vi "Read Global Header.vi"(8 "error in (no error)":errorcluster, 11 "pcap Parse and Build in":refnum<class "pcap Parse and Build.lvclass">) -> (0 "error out":errorcluster, 2 "Global Header":T1={"magic number"=2712812621, "Major Version"=2, "Minor Version"=4, "This Zone"=0, "Accuracy"=0, "Max Length"=65535, "Data Link"=1} {"magic number" format="%.0x"}, 3 "pcap Parse and Build out":refnum<class "pcap Parse and Build.lvclass">)   [LabVIEW 2021, in "pcap Parse and Build.lvclass"]
uses:
  pcap Parse and Build.lvclass
  Typedef/Global Header.ctl
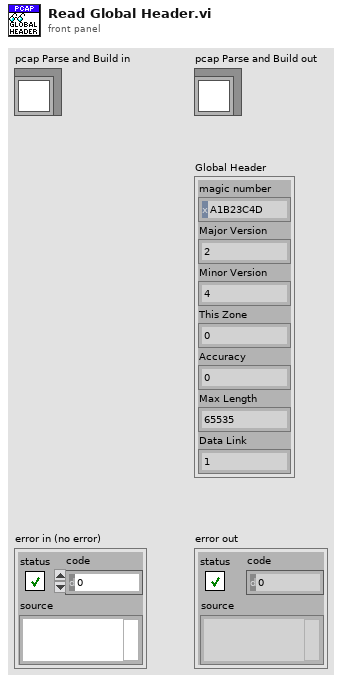
[diagram p1: front panel]
types:
  T1 = typedef "pcap Parse and Build.lvclass/Global Header.ctl" = cluster{"magic number":u32, "Major Version":u16, "Minor Version":u16, "This Zone":u32, "Accuracy":u32, "Max Length":u32, "Data Link":u32}
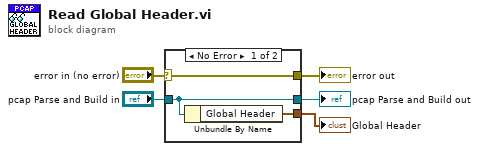
[diagram p0: block diagram]
diagram:
  n1 = case shown="No Error" "error in (no error)" {
    selector: "error in (no error)" -> [w8 w9]
    tunnel: [w8 w9] -> w4
    tunnel: [w7 w10] -> w2
    tunnel: "pcap Parse and Build in" -> [w7 w10]
    tunnel: [w6 _] -> w1
    frame No Error {
      n2 = Unbundle By Name(w7) -> ("Global Header"=w6:T1)
    }
    frame Error {
    }
  }
  "error out" <- w4
  "pcap Parse and Build out" <- w2
  "Global Header" <- w1
